vi "Notify Launcher.vi"(8 "error in (no error)":errorcluster, 9 "milliseconds to wait":u32, 10 "Notification":string, 11 "Application Controller in":refnum<class "Application Controller.lvclass">) -> (0 "error out":errorcluster, 3 "Application Controller out":refnum<class "Application Controller.lvclass">)   [LabVIEW 2024, in "Application Controller.lvclass"]
uses:
  Application Controller.lvclass
  Application Controller.lvclass/Application Controller.ctl
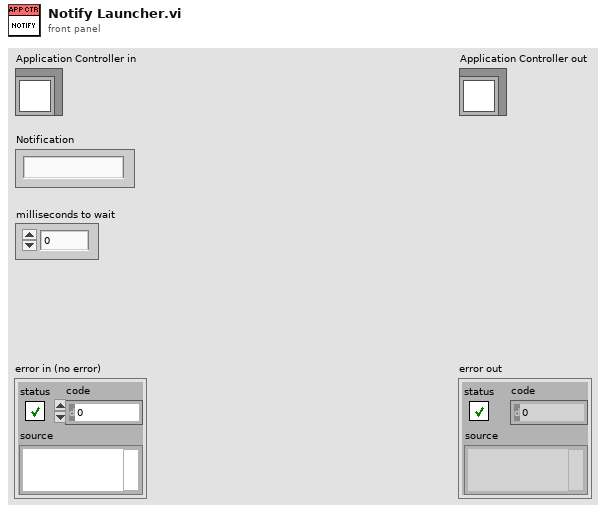
[diagram p1: front panel]
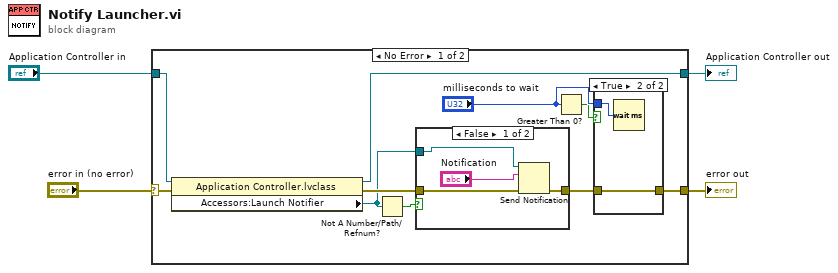
[diagram p0: block diagram]
diagram:
  n1 = case shown="No Error" "error in (no error)" {
    selector: "error in (no error)" -> [w13 w24]
    tunnel: [w11 w24] -> w3
    tunnel: [w6 w23] -> w1
    tunnel: "Application Controller in" -> [w7 w23]
    frame No Error {
      n2 = property class="Application Controller.lvclass"(reference=w7, error in=w13) -> (reference out=w6:refnum<class "Application Controller.lvclass">, error out=w8:errorcluster, "Accessors:Launch Notifier"=w5:refnum<notifier>)
      n3 = Not A Number/Path/Refnum?(number/path/refnum=w5) -> (NaN/Path/Refnum?=w14:bool)
      n4 = case shown="False" w14 {
        tunnel: w5 -> [w20 _]
        tunnel: w8 -> [w19 w22]
        tunnel: [w18 w22] -> w12
        frame False {
          n5 = Send Notification(notification="Notification", notifier=w20, error in (no error)=w19) -> (error out=w18:errorcluster)  [unwired: 1 out]
        }
        frame True {
        }
      }
      n6 = Greater Than 0?(x="milliseconds to wait") -> (x > 0?=w9:bool)
      n7 = case shown="True" w9 {
        tunnel: "milliseconds to wait" -> [_ w17]
        tunnel: w12 -> [w15 w16]
        tunnel: [w15 w16] -> w11
        frame False {
        }
        frame True {
          n8 = Wait (ms)(milliseconds to wait=w17) -> ()  [unwired: 1 out]
        }
      }
    }
    frame Error {
    }
  }
  "error out" <- w3
  "Application Controller out" <- w1
